vi "4155C SampleI Config SMUs v3.0.vi"(4 "Sample I - Probe 4 (Disabled)":u32(ring)=3 items=["SMU1  ", "SMU2  ", "SMU3  ", "SMU4  ", "SMU5  ", "SMU6  ", "VSU1  ", "VSU2  "], 5 "Sample I - Drain/Gate":u32(ring)=1 items=["SMU1  ", "SMU2  ", "SMU3  ", "SMU4  ", "SMU5  ", "SMU6  ", "VSU1  ", "VSU2  "], 6 "Sample I - Probe 3 (Disabled)":u32(ring)=2 items=["SMU1  ", "SMU2  ", "SMU3  ", "SMU4  ", "SMU5  ", "SMU6  ", "VSU1  ", "VSU2  "], 7 "Sample I - Source/Common":u32(ring) items=["SMU1  ", "SMU2  ", "SMU3  ", "SMU4  ", "SMU5  ", "SMU6  ", "VSU1  ", "VSU2  "], 8 "error in (no error)":errorcluster, 9 "Gate Standby":bool, 10 "Drain Standby":bool, 11 "VISA resource name in":refnum<visa-resource-name>) -> (0 "error out":errorcluster, 3 "VISA Resource Name out":refnum<visa-resource-name>)   [LabVIEW 2016]
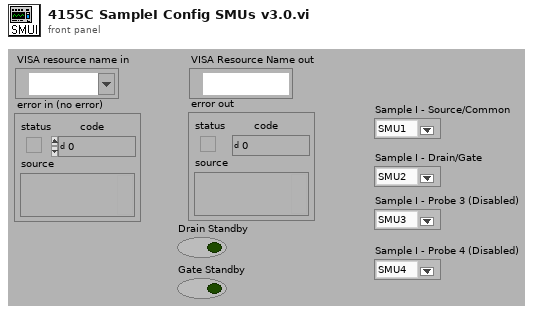
[diagram p1: front panel]
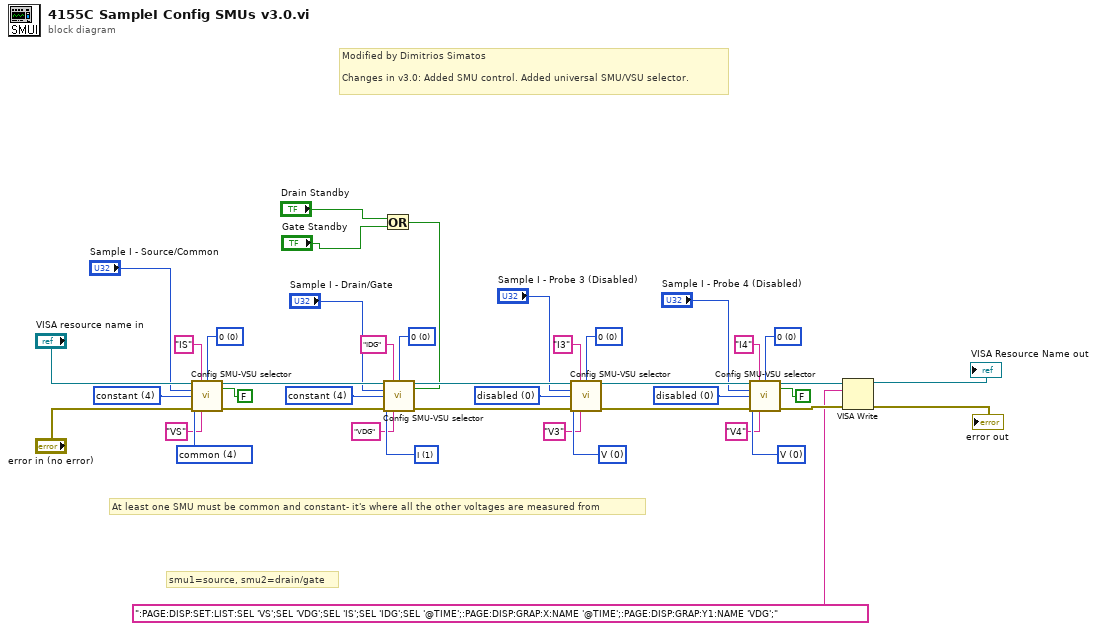
[diagram p0: block diagram]
diagram:
  w21 = u32 0 items=["V  ", "I  ", "V pulse  ", "I pulse  ", "  common  "] ("mode")
  w22 = u32 0 items=["0  ", "10K Ohms  ", "100K Ohms  ", "1M Ohms  "] ("series resistance *")
  w24 = u32 0 items=["disabled  ", "VAR1  ", "VAR2  ", "VAR1'  ", "constant  "] ("function")
  w26 = u32 0 items=["V  ", "I  ", "V pulse  ", "I pulse  ", "  common  "] ("mode")
  w27 = u32 0 items=["0  ", "10K Ohms  ", "100K Ohms  ", "1M Ohms  "] ("series resistance *")
  w29 = u32 0 items=["disabled  ", "VAR1  ", "VAR2  ", "VAR1'  ", "constant  "] ("function")
  w31 = u32 1 items=["V  ", "I  ", "V pulse  ", "I pulse  ", "  common  "] ("mode")
  w32 = u32 0 items=["0  ", "10K Ohms  ", "100K Ohms  ", "1M Ohms  "] ("series resistance *")
  w34 = u32 4 items=["disabled  ", "VAR1  ", "VAR2  ", "VAR1'  ", "constant  "] ("function")
  w37 = u32 4 items=["V  ", "I  ", "V pulse  ", "I pulse  ", "  common  "] ("mode")
  w38 = u32 0 items=["0  ", "10K Ohms  ", "100K Ohms  ", "1M Ohms  "] ("series resistance *")
  w40 = u32 4 items=["disabled  ", "VAR1  ", "VAR2  ", "VAR1'  ", "constant  "] ("function")
  # "Modified by Dimitrios Simatos\n\nChanges in v3.0: Added SMU control. Added universal SMU/VSU selector."
  # "smu1=source, smu2=drain/gate"
  # "At least one SMU must be common and constant- it's where all the other voltages are measured from"
  n1 = call "Config SMU-VSU selector.vi"("VISA session"="VISA resource name in", "I name (max 6 chars)"="IS", "standby"=FALSE, "unit to configure"="Sample I - Source/Common", "function"=w40, "mode"=w37, "error in (no error)"="error in (no error)", "V name (max 6 chars)"="VS", "series resistance *"=w38) -> ("dup VISA resource name"=w18:refnum<visa-resource-name>, "error out"=w17:errorcluster)  [unwired: 3 in, 2 out]
  n2 = Or(x="Drain Standby", y="Gate Standby") -> (x .or. y?=w5:bool)
  n3 = call "Config SMU-VSU selector.vi"("VISA session"=w18, "I name (max 6 chars)"="IDG", "standby"=w5, "unit to configure"="Sample I - Drain/Gate", "function"=w34, "mode"=w31, "error in (no error)"=w17, "V name (max 6 chars)"="VDG", "series resistance *"=w32) -> ("dup VISA resource name"=w15:refnum<visa-resource-name>, "error out"=w16:errorcluster)  [unwired: 3 in, 2 out]
  n4 = call "Config SMU-VSU selector.vi"("VISA session"=w15, "I name (max 6 chars)"="I3", "unit to configure"="Sample I - Probe 3 (Disabled)", "function"=w29, "mode"=w26, "error in (no error)"=w16, "V name (max 6 chars)"="V3", "series resistance *"=w27) -> ("dup VISA resource name"=w14:refnum<visa-resource-name>, "error out"=w13:errorcluster)  [unwired: 4 in, 2 out]
  n5 = call "Config SMU-VSU selector.vi"("VISA session"=w14, "I name (max 6 chars)"="I4", "standby"=FALSE, "unit to configure"="Sample I - Probe 4 (Disabled)", "function"=w24, "mode"=w21, "error in (no error)"=w13, "V name (max 6 chars)"="V4", "series resistance *"=w22) -> ("dup VISA resource name"=w12:refnum<visa-resource-name>, "error out"=w11:errorcluster)  [unwired: 3 in, 2 out]
  n6 = VISA Write(VISA resource name=w12, write buffer=":PAGE:DISP:SET:LIST:SEL 'VS';SEL 'VDG';SEL 'IS';SEL 'IDG';SEL '@TIME';:PAGE:DISP:GRAP:X:NAME '@TIME';:PAGE:DISP:GRAP:Y1:NAME 'VDG';" ("write buffer (\"\")"), error in (no error)=w11) -> (VISA resource name out=→"VISA Resource Name out":refnum<visa-resource-name>, error out=→"error out":errorcluster)  [unwired: 1 out]
